vi "Configure Standard Waveform Advanced.vi"   [LabVIEW 2015, in "Agilent 3352X Series.lvlib"]
doc: "Configure some specific settings for standard waveform function like Ramp, Square and Pulse."
uses:
  <instrlib>/Agilent 3352X Series/Agilent 3352X Series.lvlib
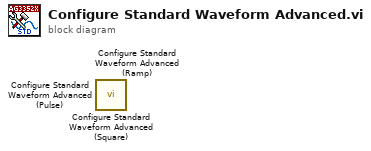
[diagram p0: block diagram]
diagram:
  n1 = call <instrlib>:"Configure Standard Waveform Advanced (Square).vi"() -> ()  [unwired: 10 in, 2 out]
  n2 = call <instrlib>:"Configure Standard Waveform Advanced (Ramp).vi"() -> ()  [unwired: 10 in, 2 out]
  n3 = call <instrlib>:"Configure Standard Waveform Advanced (Pulse).vi"() -> ()  [unwired: 10 in, 2 out]
